vi "All Interediate Structures.vi"(4 "Collision Radius (A)":dbl=2.0, 6 "Avoid Collision":bool, 8 "Map back to [0,1) ?":bool, 9 "Second Structure":T1, 10 "First Structure":T1, 11 "# Frames":i32(slide)=5 scale=0.0..100.0) -> (3 "Array of Structures":T2(array[cluster]))   [LabVIEW 2010]
uses:
  <vilib>/Analysis/_algsub.llb/Real Vector Norm.vi
  <vilib>/Analysis/NI_AALPro.lvlib
panel:
  out "System Waveform Chart":cluster{"norm":dbl, "norm":dbl, "norm":dbl}(graph)
  out "Array":cluster{"Atom Name":string, dbl[][]}[](array[cluster])
  in  "First Structure 2":T1
  in  "Second Structure 2":T1
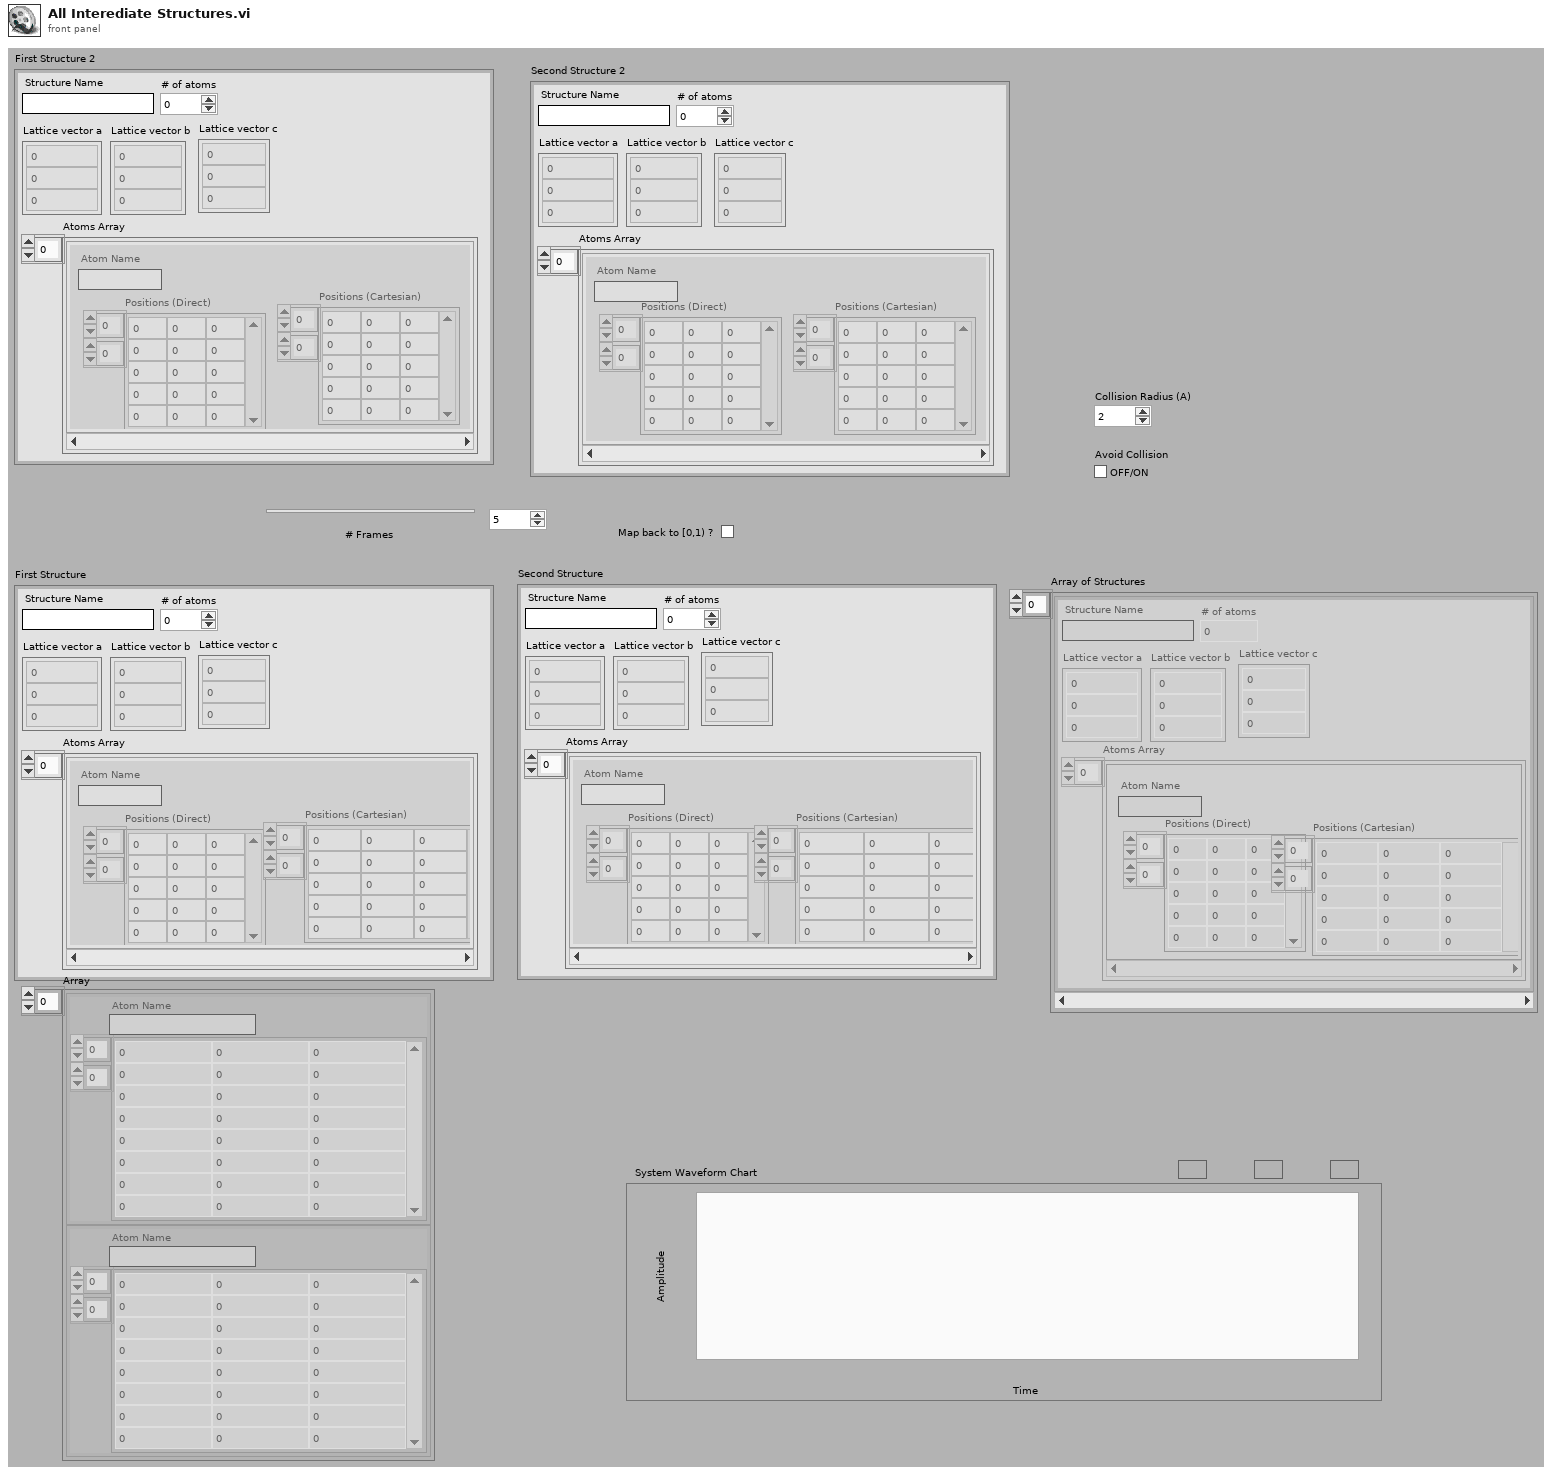
[diagram p1: front panel]
types:
  T1 = cluster{"Structure Name":string, "Lattice vector a":dbl[], "Lattice vector b":dbl[], "Lattice vector c":dbl[], "Atoms Array":cluster{"Atom Name":string, "Positions (Direct)":dbl[][], "Positions (Cartesian)":dbl[][]}[], "# of atoms":i32}
  T2 = cluster{"Structure Name":string, "Lattice vector a":dbl[], "Lattice vector b":dbl[], "Lattice vector c":dbl[], "Atoms Array":cluster{"Atom Name":string, "Positions (Direct)":dbl[][], "Positions (Cartesian)":dbl[][]}[], "# of atoms":i32}[]
  T3 = cluster{"Atom Name":string, "Positions (Direct)":dbl[][], "Positions (Cartesian)":dbl[][]}[]
  T4 = cluster{"Atom Name":string, "Positions (Direct)":dbl[][], dbl[][]}
  T5 = cluster{"Structure ID":string, "Lattice vector a":dbl[], "Lattice vector b":dbl[], "Lattice vector c":dbl[], "Atoms Array":cluster{"Atom Name":string, "Positions (Direct)":dbl[][], "Positions (Cartesian)":dbl[][]}[], "# of atoms":i32}
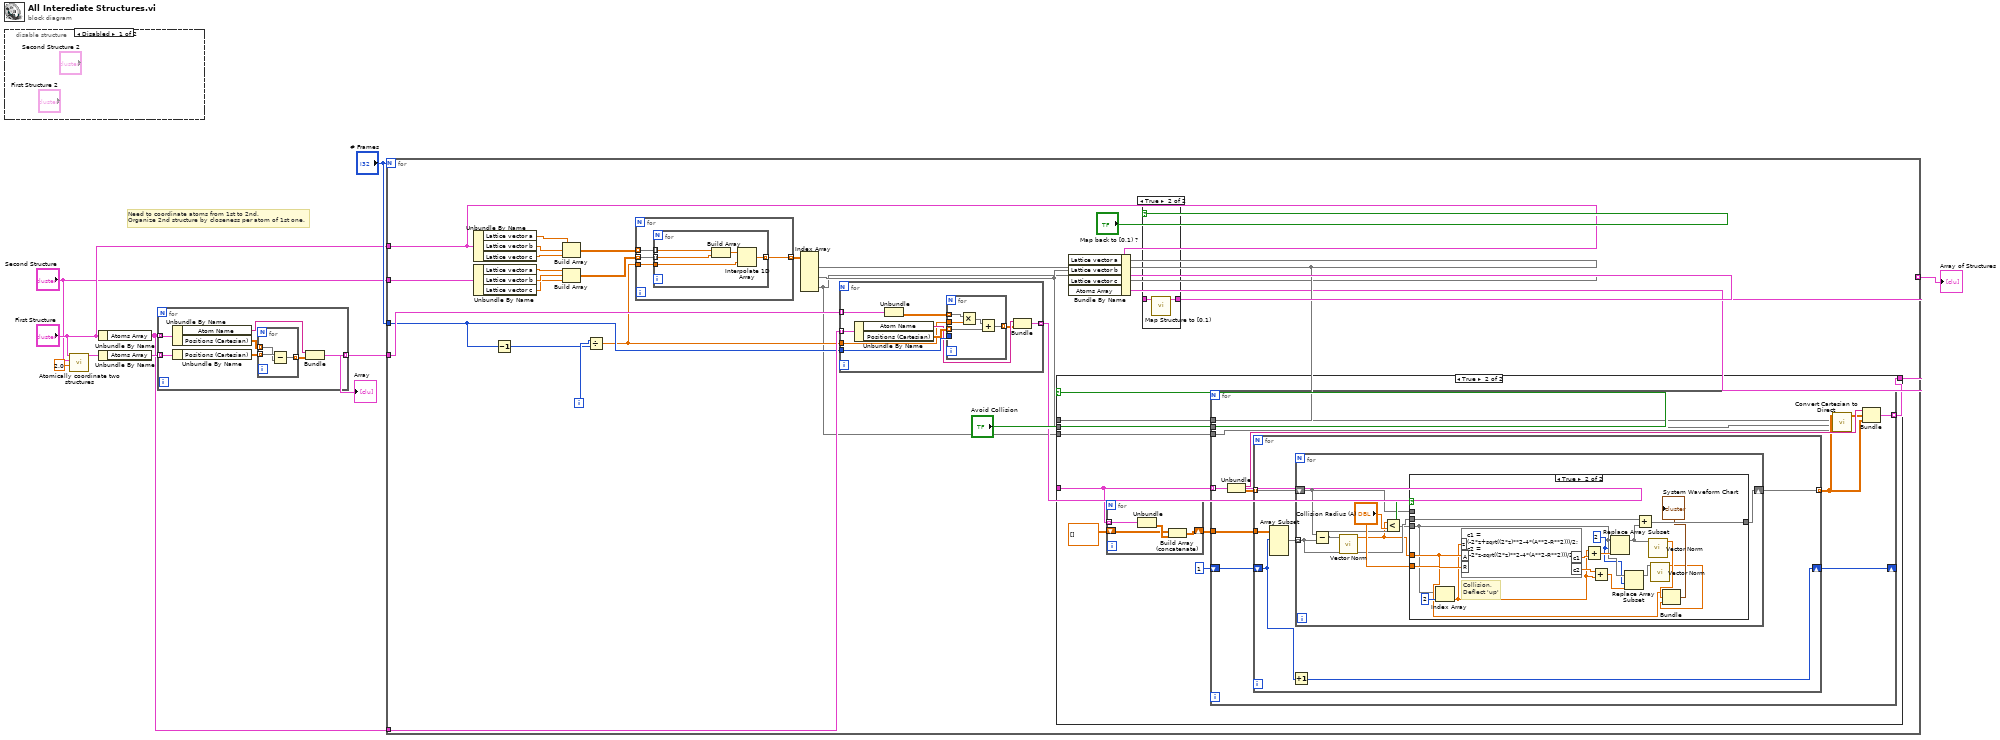
[diagram p0: block diagram]
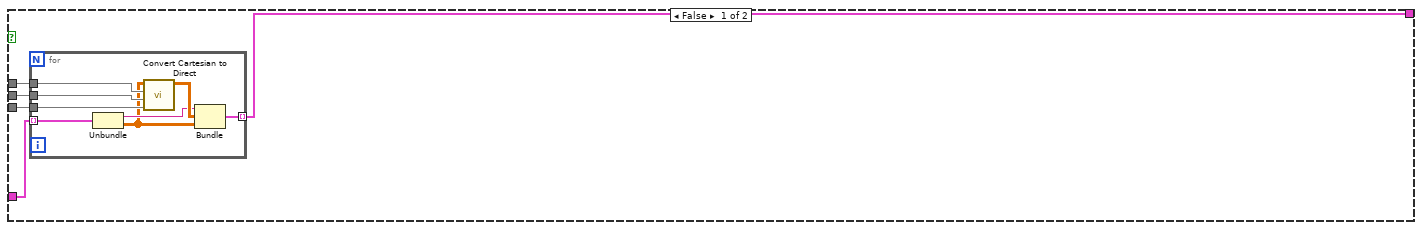
[diagram p3: hidden frame]
diagram:
  # "Need to coordinate atoms from 1st to 2nd.\nOrganize 2nd structure by closeness per atom of 1st one."
  n1 = disable-structure shown="Disabled" {
    frame Disabled {
    }
    frame Enabled {
    }
  }
  n2 = call "Atomically coordinate two structures.vi"("1st Pass Closeness"=2.0, "Second Structure"="Second Structure", "First Structure"="First Structure") -> ("Coordinated 2nd Structure"=w3:T1)  [unwired: 8 in]
  n3 = Unbundle By Name("First Structure") -> ("Atoms Array"=w7:T3)
  n4 = Unbundle By Name(w3) -> ("Atoms Array"=w9:T3)
  n5 = for {
    tunnel: w7 -> [w16] mode=indexing
    tunnel: w9 -> [w15] mode=indexing
    tunnel: [w12] -> w8 mode=indexing
    n6 = Unbundle By Name(w16) -> ("Atom Name"=w14:string, "Positions (Cartesian)"=w10:dbl[][])
    n7 = Unbundle By Name(w15) -> ("Positions (Cartesian)"=w11:dbl[][])
    n8 = for {
      tunnel: w10 -> [w18] mode=indexing
      tunnel: w11 -> [w19] mode=indexing
      tunnel: [w17] -> w13 mode=indexing
      n9 = Subtract(x=w19, y=w18) -> (x-y=w17:dbl[])
    }
    n10 = Bundle("Atom Name"=w14, w13) -> (w12:cluster{"Atom Name":string, dbl[][]})  [unwired: 1 in]
  }
  "Array" <- w8
  n11 = for {
    N: "# Frames" -> [_]
    tunnel: w8 -> [w45]
    tunnel: w7 -> [w44]
    tunnel: "First Structure" -> [w37]
    tunnel: [w39] -> w5 mode=indexing
    tunnel: "# Frames" -> [w42]
    tunnel: "Second Structure" -> [w36]
    i -> [w43]
    n12 = Unbundle By Name(w37) -> ("Lattice vector a"=w35:dbl[], "Lattice vector b"=w34:dbl[], "Lattice vector c"=w33:dbl[])
    n13 = Unbundle By Name(w36) -> ("Lattice vector a"=w32:dbl[], "Lattice vector b"=w31:dbl[], "Lattice vector c"=w30:dbl[])
    n14 = Decrement(x=w42) -> (x-1=w41:i32)
    n15 = Build Array(w35, w34, w33) -> (w29:dbl[][])
    n16 = Build Array(w32, w31, w30) -> (w28:dbl[][])
    n17 = Divide(x=w43, y=w41) -> (x/y=w27:dbl)
    n18 = for {
      tunnel: w29 -> [w117] mode=indexing
      tunnel: w28 -> [w116] mode=indexing
      tunnel: [w115] -> w26 mode=indexing
      tunnel: w27 -> [w114]
      n19 = for {
        tunnel: w117 -> [w122] mode=indexing
        tunnel: w116 -> [w121] mode=indexing
        tunnel: [w119] -> w115 mode=indexing
        tunnel: w114 -> [w118]
        n20 = Build Array(w122, w121) -> (w120:dbl[])
        n21 = Interpolate 1D Array(1:w118, 2:w120) -> (0:w119:dbl)
      }
    }
    n22 = Index Array(array=w26) -> (element #1=w23:dbl[], element #2=w22:dbl[], element #3=w21:dbl[])  [unwired: 6 in]
    n23 = for {
      tunnel: w45 -> [w133] mode=indexing
      tunnel: w44 -> [w134] mode=indexing
      tunnel: w42 -> [w130]
      tunnel: [w128] -> w24 mode=indexing
      tunnel: w27 -> [w127]
      n24 = Unbundle By Name(w134) -> ("Atom Name"=w129:string, "Positions (Cartesian)"=w132:dbl[][])
      n25 = Unbundle(w133) -> (w131:dbl[][])  [unwired: 1 out]
      n26 = for {
        tunnel: w132 -> [w139] mode=indexing
        tunnel: w131 -> [w138] mode=indexing
        tunnel: w130 -> [_]
        tunnel: [w136] -> w126 mode=indexing
        tunnel: w127 -> [w135]
        n27 = Multiply(x=w138, y=w135) -> (x*y=w137:dbl[])
        n28 = Add(x=w137, y=w139) -> (x+y=w136:dbl[])
      }
      n29 = Bundle("Atom Name"=w129, w126) -> (w128:cluster{"Atom Name":string, dbl[][]})  [unwired: 1 in]
    }
    n30 = case shown="True" "Avoid Collision" {
      tunnel: w24 -> [w50 w64]
      tunnel: w23 -> [w49 w61]
      tunnel: w22 -> [w48 w60]
      tunnel: w21 -> [w47 w59]
      tunnel: [w46 w62] -> w20
      frame False {
        n31 = for {
          tunnel: w50 -> [w58] mode=indexing
          tunnel: w49 -> [w57]
          tunnel: w48 -> [w56]
          tunnel: w47 -> [w55]
          tunnel: [w51] -> w46 mode=indexing
          n32 = Unbundle(w58) -> ("Atom Name"=w53:string, w52:dbl[][])
          n33 = call "Convert Cartesian to Direct.vi"("Lattice vector c"=w55, "Lattice vector b"=w56, "Lattice vector a"=w57, "Positions (Cartesian)"=w52) -> ("Positions (Direct)"=w54:dbl[][])  [unwired: 7 in]
          n34 = Bundle("Atom Name"=w53, "Positions (Direct)"=w54, w52) -> (w51:T4)  [unwired: 1 in]
        }
      }
      frame True {
        n35 = for {
          tunnel: w64 -> [w113] mode=indexing
          shift-right: [w111] -> w65
          shift-left: dbl[][] [] -> [w110]
          n36 = Unbundle(w113) -> (w112:dbl[][])  [unwired: 1 out]
          n37 = Build Array (concatenate)(w110, w112) -> (w111:dbl[][])
        }
        n38 = for {
          tunnel: w65 -> [w78]
          tunnel: w64 -> [w77] mode=indexing
          shift-right: [w75] -> _
          shift-left: 1 -> [w74]
          tunnel: [w71] -> w62 mode=indexing
          tunnel: w61 -> [w69]
          tunnel: w60 -> [w68]
          tunnel: w59 -> [w67]
          n39 = Unbundle(w77) -> ("Atom Name"=w73:string, w76:dbl[][])
          n40 = for {
            tunnel: w76 -> [w82] mode=indexing
            tunnel: w78 -> [w84]
            tunnel: [w81] -> w70 mode=indexing
            shift-right: [w79] -> w75
            shift-left: w74 -> [w80]
            n41 = Array Subset(array=w84, index (row)=w80) -> (w83:dbl[][])  [unwired: 3 in]
            n42 = Increment(x=w80) -> (x+1=w79:i32)
            n43 = for {
              tunnel: w83 -> [w88] mode=indexing
              shift-right: [w90] -> w81
              shift-left: w82 -> [w86]
              n44 = Subtract(x=w86, y=w88) -> (x-y=w87:dbl[])
              n45 = call-poly <vilib>:"Vector Norm.vi"("Input Vector"=w87) -> ("norm"=w85:dbl)  [unwired: 9 in, 1 out]
              n46 = Less?(x=w85, y="Collision Radius (A)") -> (x < y?=w91:bool)
              n47 = case shown="True" w91 {
                tunnel: [w92 w105] -> w90
                tunnel: w87 -> [_ w97]
                tunnel: w85 -> [_ w102]
                tunnel: "Collision Radius (A)" -> [_ w108]
                tunnel: w88 -> [_ w106]
                tunnel: w86 -> [w92 _]
                frame False {
                }
                frame True {
                  w95 = 2 ("index")
                  # "Collision,\nDeflect 'up'"
                  n48 = Index Array(array=w97, index=2) -> (element=w99:dbl)
                  n49 = formula code="c1 = (-2*z+sqrt((2*z)**2-4*(A**2-R**2)))/2;\nc2 = (-2*z-sqrt((2*z)**2-4*(A**2-R**2)))/2;"("z"=w99, "A"=w102, "R"=w108) -> ("c1"=w107:dbl, "c2"=w100:dbl)
                  n50 = Add(x=w99, y=w107) -> (x+y=w98:dbl)
                  n51 = Add(x=w100, y=w99) -> (x+y=w96:dbl)
                  n52 = Replace Array Subset(array=w97, new element=w98, index=w95) -> (w104:dbl[])
                  n53 = Replace Array Subset(array=w97, new element=w96, index=w95) -> (w94:dbl[])
                  n54 = Add(x=w106, y=w104) -> (x+y=w105:dbl[])
                  n55 = call-poly <vilib>:"Vector Norm.vi"("Input Vector"=w104) -> ("norm"=w103:dbl)  [unwired: 9 in, 1 out]
                  n56 = call-poly <vilib>:"Vector Norm.vi"("Input Vector"=w94) -> ("norm"=w93:dbl)  [unwired: 9 in, 1 out]
                  n57 = Bundle("norm"=w102, "norm"=w103, "norm"=w93) -> (→"System Waveform Chart":cluster{"norm":dbl, "norm":dbl, "norm":dbl})  [unwired: 1 in]
                }
              }
            }
          }
          n58 = call "Convert Cartesian to Direct.vi"("Lattice vector c"=w67, "Lattice vector b"=w68, "Lattice vector a"=w69, "Positions (Cartesian)"=w70) -> ("Positions (Direct)"=w72:dbl[][])  [unwired: 7 in]
          n59 = Bundle("Atom Name"=w73, "Positions (Direct)"=w72, w70) -> (w71:T4)  [unwired: 1 in]
        }
      }
    }
    n60 = Bundle By Name(cluster=w37, "Lattice vector a"=w23, "Lattice vector b"=w22, "Lattice vector c"=w21, "Atoms Array"=w20) -> (w40:T1)
    n61 = case shown="True" "Map back to [0,1) ?" {
      tunnel: w40 -> [w123 w125]
      tunnel: [w123 w124] -> w39
      frame False {
      }
      frame True {
        n62 = call "Map Structure to [0,1).vi"("Structure"=w125) -> ("Structure mapped to [0,1)"=w124:T5)  [unwired: 10 in]
      }
    }
  }
  "Array of Structures" <- w5
